vi "Corners to Rectangle.vi"(10 "Corners 2":cluster{"X":sgl, "Y":sgl}[](array[cluster])=[{"X"=418.12665, "Y"=424.52673}, {"X"=459.83737, "Y"=432.6989}, {"X"=455.7626, "Y"=481.78384}, {"X"=413.9875, "Y"=474.98163}, {"X"=418.12665, "Y"=424.52673}]) -> (2 "output cluster":T2, 4 "Aspect Ratio":sgl, 5 "Center":cluster{"X":dbl, "Y":dbl} {"Y" format="%0.2f"; "X" format="%0.2f"}, 6 "AprilTag Location":T1 {"Rotation" format="%.2f"; "Left" scale=0.0..1024.0; "Right" scale=0.0..1024.0})   [LabVIEW 2023]
uses:
  Target Fields.ctl
  <vilib>/Analysis/baseanly.llb/Mean (DBL).vi
  <vilib>/Analysis/NI_AALBase.lvlib
panel:
  out "Tilted Left/Right":bool
  out "Tilted Up/down":bool
  out "Vert Size":sgl
  out "Horz Size":sgl
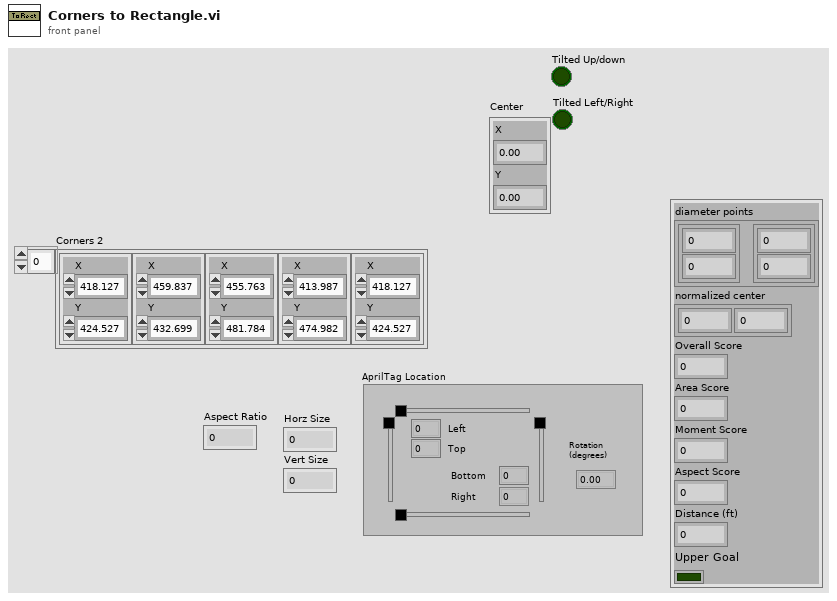
[diagram p1: front panel]
types:
  T1 = typedef "IMAQ Rectangle" = cluster{"Left":i32, "Top":i32, "Right":i32, "Bottom":i32, "Rotation":dbl}
  T2 = typedef "Target Fields.ctl" = cluster{"diameter points":cluster{"first point":cluster{"x":dbl, "y":dbl}, "projected point":cluster{"x":dbl, "y":dbl}}, "normalized center":cluster{"x":dbl, "y":dbl}, "Overall Score":dbl, "Area Score":dbl, "Moment Score":dbl, "Aspect Score":dbl, "Distance (ft)":dbl, "Upper Goal":bool}
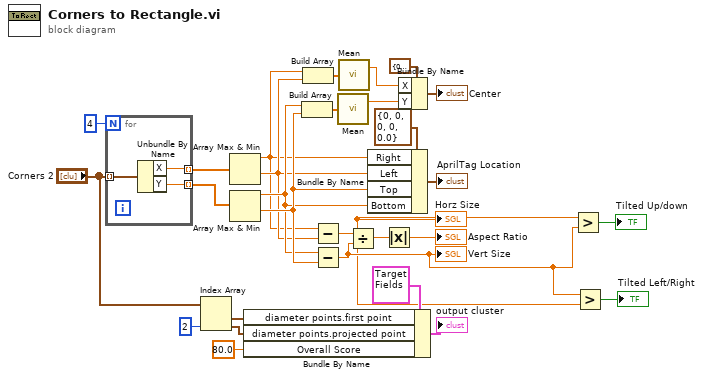
[diagram p0: block diagram]
diagram:
  n1 = for {
    N: 4 -> [_]
    tunnel: "Corners 2" -> [w31] mode=indexing
    tunnel: [w30] -> w28 mode=indexing
    tunnel: [w29] -> w27 mode=indexing
    n2 = Unbundle By Name(w31) -> ("X"=w30:sgl, "Y"=w29:sgl)
  }
  n3 = Index Array(array="Corners 2", index #2=2 ("index")) -> (element #1=w15:cluster{"X":sgl, "Y":sgl}, element #2=w14:cluster{"X":sgl, "Y":sgl})  [unwired: 1 in]
  n4 = Array Max & Min(array=w28) -> (max value=w1:sgl, min value=w2:sgl)  [unwired: 2 out]
  n5 = Array Max & Min(array=w27) -> (max value=w3:sgl, min value=w4:sgl)  [unwired: 2 out]
  n6 = Bundle By Name(cluster=T2 {"diameter points"={"first point"={"x"=0.0, "y"=0.0}, "projected point"={"x"=0.0, "y"=0.0}}, "normalized center"={"x"=0.0, "y"=0.0}, "Overall Score"=0.0, "Area Score"=0.0, "Moment Score"=0.0, "Aspect Score"=0.0, "Distance (ft)"=0.0, "Upper Goal"=FALSE} ("results"), "diameter points.first point"=w15, "diameter points.projected point"=w14, "Overall Score"=80.0) -> (→"output cluster":T2)
  n7 = Build Array(w3, w4) -> (w22:sgl[])
  n8 = Build Array(w1, w2) -> (w23:sgl[])
  n9 = Subtract(x=w1, y=w2) -> (x-y=w7:sgl)
  "Horz Size" <- w7
  n10 = Subtract(x=w3, y=w4) -> (x-y=w8:sgl)
  "Vert Size" <- w8
  n11 = call-poly <vilib>:"Mean.vi"("X"=w22) -> ("mean"=w19:dbl)  [unwired: 1 out]
  n12 = call-poly <vilib>:"Mean.vi"("X"=w23) -> ("mean"=w20:dbl)  [unwired: 1 out]
  n13 = Divide(x=w7, y=w8) -> (x/y=w25:sgl)
  n14 = Bundle By Name(cluster=T1 {"Left"=0, "Top"=0, "Right"=0, "Bottom"=0, "Rotation"=0.0} ("Rectangle"), "Right"=w1, "Left"=w2, "Top"=w4, "Bottom"=w3) -> (→"AprilTag Location":T1)
  n15 = Absolute Value(x=w25) -> (abs(x)=→"Aspect Ratio":sgl)
  n16 = Bundle By Name(cluster=cluster{"X":dbl, "Y":dbl} {"X"=0.0, "Y"=0.0} ("Center"), "X"=w20, "Y"=w19) -> (→"Center":cluster{"X":dbl, "Y":dbl})
  n17 = Greater?(x=w7, y=w8) -> (0:→"Tilted Up/down":bool)
  n18 = Greater?(x=w8, y=w7) -> (0:→"Tilted Left/Right":bool)
